vi "Clear.vi"(8 "error in (no error)":errorcluster, 11 "Normal Log in":refnum<class "Normal Log.lvclass">) -> (0 "error out":errorcluster, 3 "Normal Log out":refnum<class "Normal Log.lvclass">)   [LabVIEW 2020, in "Normal Log.lvlib" / "Normal Log.lvclass"]
uses:
  Normal Log.lvclass
  Normal Log Messages/Clear Log Msg/Clear Log Msg.lvclass
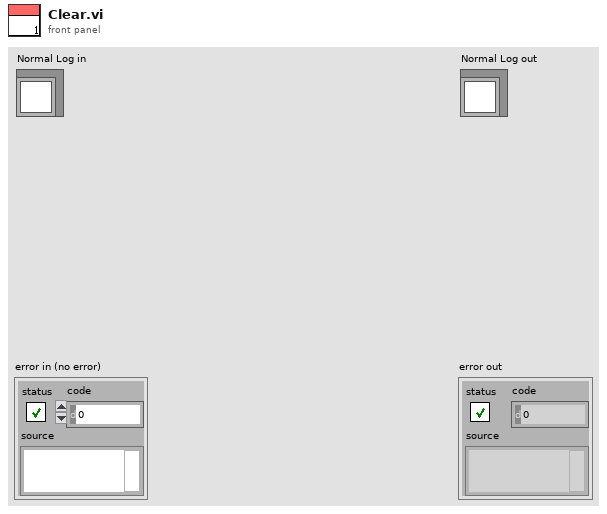
[diagram p1: front panel]
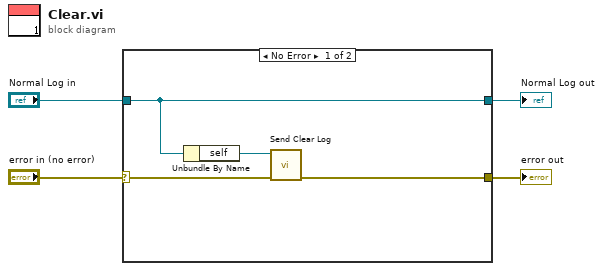
[diagram p0: block diagram]
diagram:
  n1 = case shown="No Error" "error in (no error)" {
    selector: "error in (no error)" -> [w7 w10]
    tunnel: [w6 w10] -> w3
    tunnel: "Normal Log in" -> [w8 w9]
    tunnel: [w8 w9] -> w1
    frame No Error {
      n2 = Unbundle By Name(w8) -> ("self"=w5:refnum<class "Message Enqueuer.lvclass">)
      n3 = call "Send Clear Log.vi"("error in (no error)"=w7, "Message Enqueuer"=w5) -> ("error out"=w6:errorcluster)  [unwired: 8 in, 1 out]
    }
    frame Error {
    }
  }
  "error out" <- w3
  "Normal Log out" <- w1
